vi "zadanie_1.vi"() -> ()   [LabVIEW 2020]
panel:
  in  "?":bool
  out "n!":dbl
  in  "n":dbl
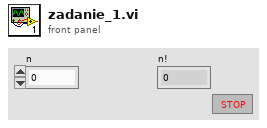
[diagram p1: front panel]
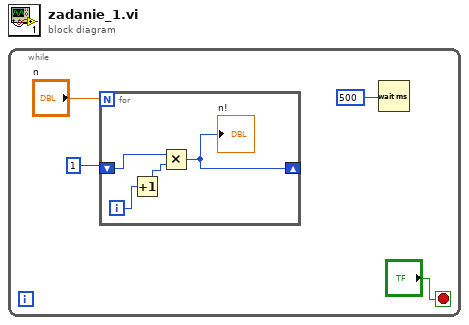
[diagram p0: block diagram]
diagram:
  n1 = while {
    stop <- "?" stop-if-true
    n2 = for {
      N: "n" -> [_]
      shift-right: [w7] -> _
      shift-left: 1 -> [w8]
      i -> [w6]
      n3 = Increment(x=w6) -> (x+1=w5:i32)
      n4 = Multiply(x=w8, y=w5) -> (x*y=w7:i32)
      "n!" <- w7
    }
    n5 = Wait (ms)(milliseconds to wait=500) -> ()  [unwired: 1 out]
  }
